vi "basic-reward.vi"(6 "Boolean":bool, 9 "Cluster 5":T1, 10 "Reward Vol. (uL)":dbl, 11 "Cluster in":refnum<vi>) -> (3 "Cluster 4":T1)   [LabVIEW 2015]
uses:
  Device/Methods/Valve-Pulse.vi
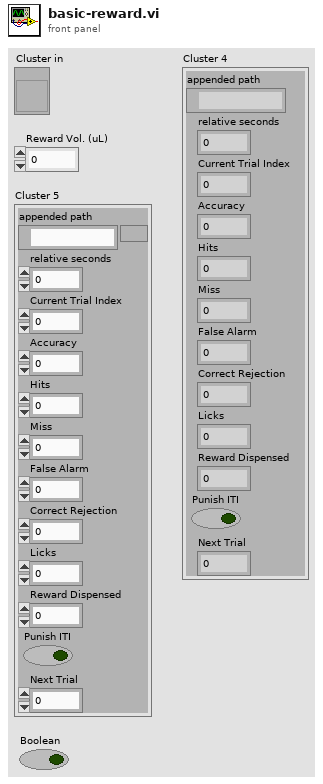
[diagram p1: front panel]
types:
  T1 = cluster{"appended path":path, "relative seconds":dbl, "Current Trial Index":i32, "Accuracy":dbl, "Hits":i32, "Miss":i32, "False Alarm":i32, "Correct Rejection":i32, "Licks":i32, "Reward Dispensed":dbl, "Punish ITI":bool, "Next Trial":i32}
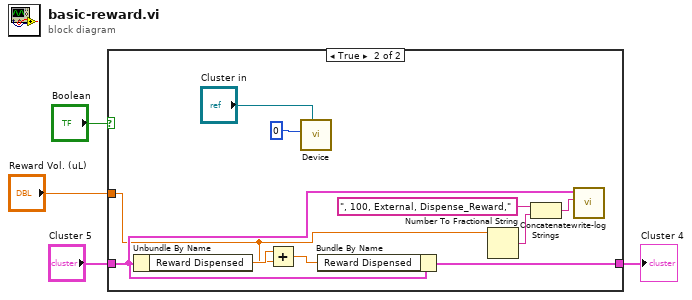
[diagram p0: block diagram]
diagram:
  n1 = case shown="True" "Boolean" {
    tunnel: "Cluster 5" -> [w5 w13]
    tunnel: [w5 w12] -> w4
    tunnel: "Reward Vol. (uL)" -> [_ w8]
    frame False {
    }
    frame True {
      n2 = Unbundle By Name(w13) -> ("Reward Dispensed"=w15:dbl)
      n3 = Add(x=w15, y=w8) -> (x+y=w14:dbl)
      n4 = call-poly "Device.vi"("Device reference"="Cluster in", "Duration"=0) -> ()  [unwired: 8 in, 2 out]
      n5 = Bundle By Name(cluster=w13, "Reward Dispensed"=w14) -> (w12:T1)
      n6 = Number To Fractional String(number=w8) -> (F-format string=w9:string)  [unwired: 3 in]
      n7 = Concatenate Strings(", 100, External, Dispense_Reward," ("text"), w9) -> (w11:string)
      n8 = call "write-log.vi"("Write Text"=w11, "Internal Cluster"=w13) -> ()  [unwired: 10 in]
    }
  }
  "Cluster 4" <- w4
